vi "Modbus.LaunchServers.vi"(8 "error in (no error)":errorcluster) -> (0 "error out":errorcluster)   [LabVIEW 2019, in "Modbus.lvlib"]
uses:
  Modbus.lvlib
  <vilib>/ni/Modbus Library/API/Wrapper/Create TCP Master.vi
  <vilib>/ni/Modbus Library/API/Master/Modbus Master.lvclass
  <vilib>/ni/Modbus Library/API/Wrapper/API Main.lvlib
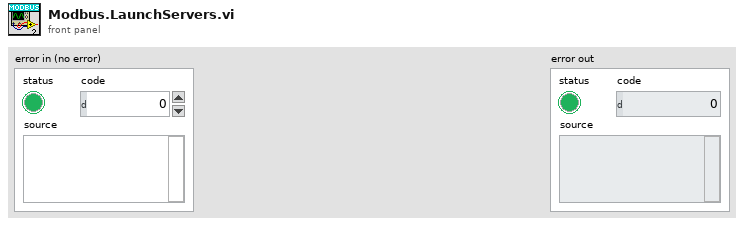
[diagram p1: front panel]
types:
  T1 = cluster{"address":string, "port (502)":u16, "connect timeout ms":i32}
  T2 = cluster{"starting address":u16, "number of inputs":u16}
  T3 = cluster{"starting address":u16, "coils to write":bool[]}
  T4 = cluster{"starting address":u16, "registers to write":u16[]}
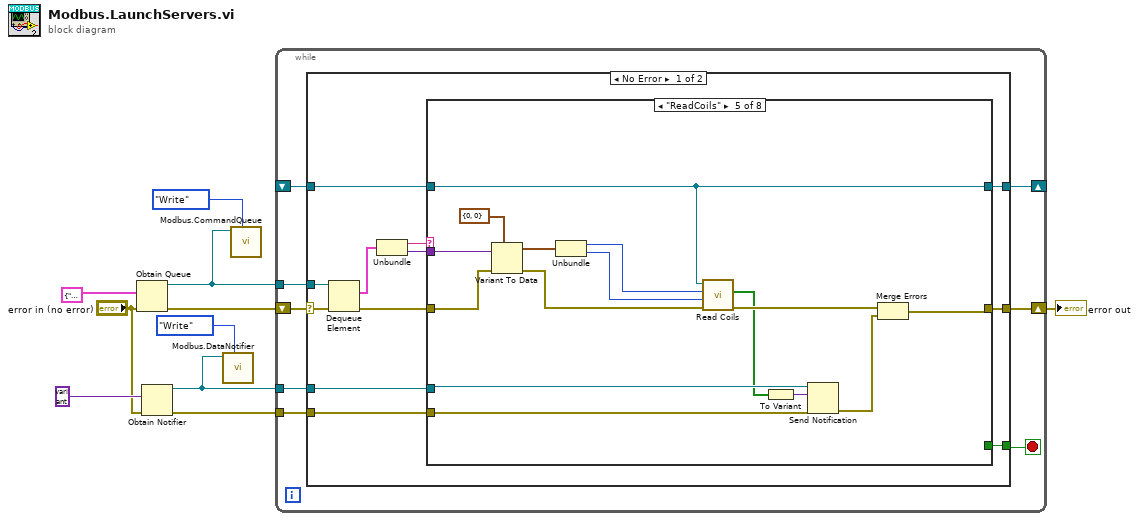
[diagram p0: block diagram]
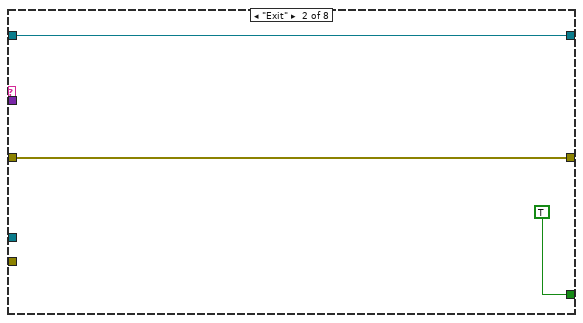
[diagram p3: hidden frame]
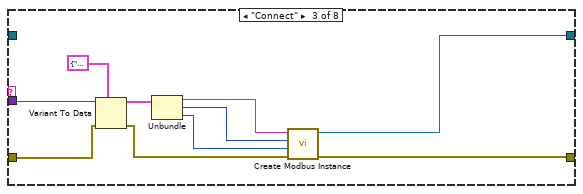
[diagram p4: hidden frame]
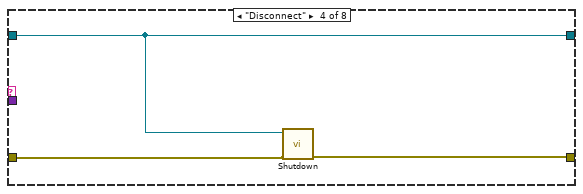
[diagram p5: hidden frame]
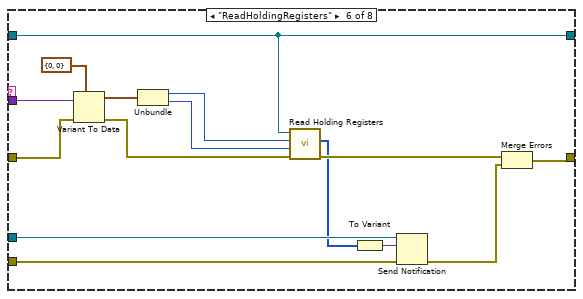
[diagram p6: hidden frame]
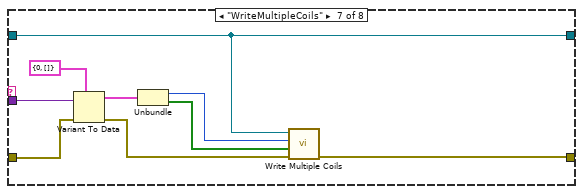
[diagram p7: hidden frame]
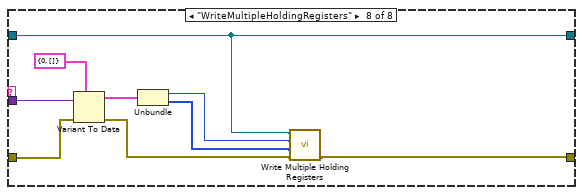
[diagram p8: hidden frame]
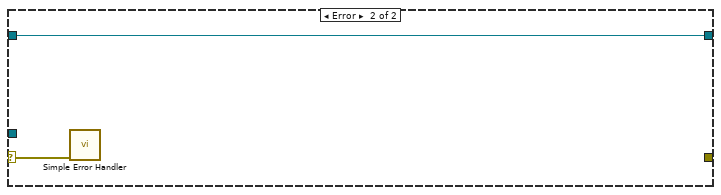
[diagram p9: hidden frame]
diagram:
  n1 = Obtain Queue(element data type=cluster{"Command":string, "Data":variant} {"Command"="", "Data"=variant}, error in (no error)="error in (no error)") -> (queue out=w6:refnum<queue>, error out=w10:errorcluster)  [unwired: 3 in, 1 out]
  n2 = Obtain Notifier(notification data type=variant, error in (no error)="error in (no error)") -> (notifier out=w4:refnum<notifier>, error out=w7:errorcluster)  [unwired: 2 in, 1 out]
  n3 = call "Modbus.DataNotifier.vi"("OP"=enum16{"Read", "Write"}."Write", "notifier IN"=w4) -> ()  [unwired: 9 in, 1 out]
  n4 = call "Modbus.CommandQueue.vi"("OP"=enum16{"Read", "Write"}."Write", "queue IN"=w6) -> ()  [unwired: 9 in, 1 out]
  n5 = while {
    tunnel: w6 -> [w17]
    shift-right: [w16] -> w2
    shift-left: w10 -> [w18]
    shift-right: [w14] -> _
    shift-left: _ -> [w13]
    tunnel: w4 -> [w12]
    tunnel: w7 -> [w11]
    stop <- w15 stop-if-true
    n6 = case shown="No Error" w18 {
      selector: w18 -> [w30 w98]
      tunnel: w17 -> [w29 _]
      tunnel: [w25 _] -> w16
      tunnel: [w23 _] -> w15
      tunnel: [w22 w97] -> w14
      tunnel: w13 -> [w21 w97]
      tunnel: w12 -> [w20 _]
      tunnel: w11 -> [w19 _]
      frame No Error {
        n7 = Dequeue Element(queue=w29, error in (no error)=w30) -> (element=w28:cluster{"Command":string, "Data":variant}, error out=w26:errorcluster)  [unwired: 1 in, 2 out]
        n8 = Unbundle(w28) -> ("Command"=w27:string, "Data"=w24:variant)
        n9 = case shown="\"ReadCoils\"" w27 {
          tunnel: w26 -> [w32 w35 w37 w48 w59 w76 w85 w94]
          tunnel: [w32 w35 w45 w47 w50 w65 w82 w91] -> w25
          tunnel: w24 -> [_ _ w43 _ w60 w77 w86 w95]
          tunnel: [_ TRUE _ _ _ _ _ _] -> w23
          tunnel: [w31 w33 w44 w46 w62 w74 w81 w90] -> w22
          tunnel: w21 -> [w31 w33 _ w46 w62 w74 w81 w90]
          tunnel: w20 -> [_ _ _ _ w54 w68 _ _]
          tunnel: w19 -> [_ _ _ _ w53 w67 _ _]
          frame Default {
          }
          frame "Exit" {
          }
          frame "Connect" {
            n10 = Variant To Data(error in=w37, type=T1 {"address"="", "port (502)"=502, "connect timeout ms"=10000}, Variant=w43) -> (data=w41:T1, error out=w36:errorcluster)
            n11 = Unbundle(w41) -> ("address"=w40:string, "port (502)"=w39:u16, "connect timeout ms"=w38:i32)
            n12 = call-poly <vilib>:"Create Modbus Instance.vi"("error in"=w36, "connect timeout ms"=w38, "port (502)"=w39, "address"=w40) -> ("error out"=w45:errorcluster, "TCP master instance"=w44:refnum<class "Modbus Master.lvclass">)  [unwired: 6 in]
          }
          frame "Disconnect" {
            n13 = call-dynamic "Shutdown.vi"("error in"=w48, "Modbus master in"=w46) -> ("error out"=w47:errorcluster)  [unwired: 9 in]
          }
          frame "ReadCoils" {
            n14 = Variant To Data(error in=w59, type=T2 {"starting address"=0, "number of inputs"=0}, Variant=w60) -> (data=w57:T2, error out=w58:errorcluster)
            n15 = Unbundle(w57) -> ("starting address"=w56:u16, "number of inputs"=w55:u16)
            n16 = call-dynamic "Read Coils.vi"("error in"=w58, "number of inputs"=w55, "starting address"=w56, "Modbus master in"=w62) -> ("error out"=w63:errorcluster, "coils"=w52:bool[])  [unwired: 5 in, 1 out]
            n17 = To Variant(anything=w52) -> (Variant=w51:variant)
            n18 = Send Notification(notification=w51, notifier=w54, error in (no error)=w53) -> (error out=w49:errorcluster)  [unwired: 1 out]
            n19 = Merge Errors(w63, w49) -> (w50:errorcluster)
          }
          frame "ReadHoldingRegisters" {
            n20 = Variant To Data(error in=w76, type=T2 {"starting address"=0, "number of inputs"=0}, Variant=w77) -> (data=w75:T2, error out=w71:errorcluster)
            n21 = Unbundle(w75) -> ("starting address"=w73:u16, "number of inputs"=w72:u16)
            n22 = call-dynamic "Read Holding Registers.vi"("error in"=w71, "number of inputs"=w72, "starting address"=w73, "Modbus master in"=w74) -> ("error out"=w70:errorcluster, "register values"=w66:u16[])  [unwired: 5 in, 1 out]
            n23 = To Variant(anything=w66) -> (Variant=w69:variant)
            n24 = Send Notification(notification=w69, notifier=w68, error in (no error)=w67) -> (error out=w64:errorcluster)  [unwired: 1 out]
            n25 = Merge Errors(w70, w64) -> (w65:errorcluster)
          }
          frame "WriteMultipleCoils" {
            n26 = Variant To Data(error in=w85, type=T3 {"starting address"=0, "coils to write"=[]}, Variant=w86) -> (data=w84:T3, error out=w83:errorcluster)
            n27 = Unbundle(w84) -> ("starting address"=w80:u16, "coils to write"=w79:bool[])
            n28 = call-dynamic "Write Multiple Coils.vi"("error in"=w83, "coils to write"=w79, "starting address"=w80, "Modbus master in"=w81) -> ("error out"=w82:errorcluster)  [unwired: 6 in, 1 out]
          }
          frame "WriteMultipleHoldingRegisters" {
            n29 = Variant To Data(error in=w94, type=T4 {"starting address"=0, "registers to write"=[]}, Variant=w95) -> (data=w93:T4, error out=w92:errorcluster)
            n30 = Unbundle(w93) -> ("starting address"=w89:u16, "registers to write"=w88:u16[])
            n31 = call-dynamic "Write Multiple Holding Registers.vi"("error in"=w92, "registers to write"=w88, "starting address"=w89, "Modbus master in"=w90) -> ("error out"=w91:errorcluster)  [unwired: 6 in, 1 out]
          }
        }
      }
      frame Error {
        n32 = call <vilib>:"Simple Error Handler.vi"("error in (no error)"=w98) -> ()  [unwired: 4 in, 5 out]
      }
    }
  }
  "error out" <- w2
